vi "transmit.vi"(8 "error in (no error)":errorcluster, 11 "M1M3SAL in":refnum<class "M1M3SAL.lvclass">) -> (0 "error out":errorcluster, 3 "M1M3SAL out":refnum<class "M1M3SAL.lvclass">)   [LabVIEW 2016, in "M1M3SupportCommunicator.lvlib" / "M1M3SAL.lvclass"]
uses:
  M1M3SAL.lvclass
  M1M3SAL.lvclass/M1M3SAL.ctl
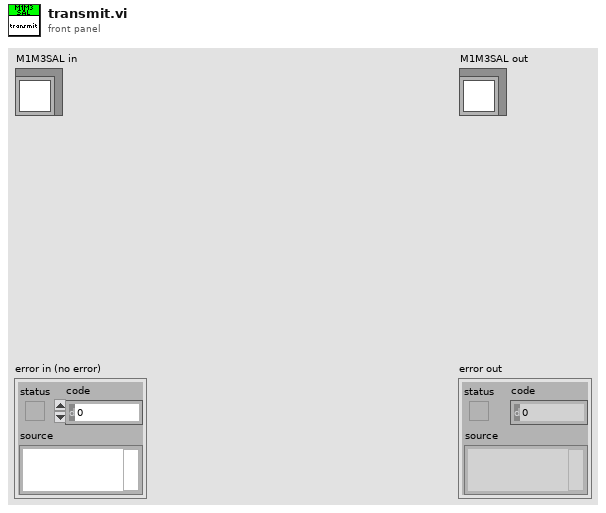
[diagram p1: front panel]
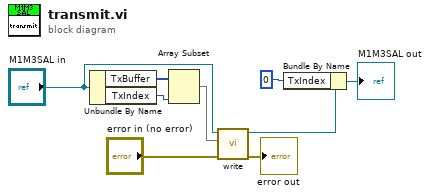
[diagram p0: block diagram]
diagram:
  n1 = Unbundle By Name("M1M3SAL in") -> ("TxBuffer"=w9:u8[], "TxIndex"=w8:i32)
  n2 = Array Subset(array=w9, length=w8) -> (w7:u8[])  [unwired: 1 in]
  n3 = call "write.vi"("error in (no error)"="error in (no error)", "Data"=w7, "M1M3SAL in"="M1M3SAL in") -> ("error out"=→"error out":errorcluster, "M1M3SAL out"=w3:refnum<class "M1M3SAL.lvclass">)  [unwired: 7 in]
  n4 = Bundle By Name(cluster=w3, "TxIndex"=0) -> (→"M1M3SAL out":refnum<class "M1M3SAL.lvclass">)
